vi "Create Group Transfers.vi"(7 "direction":T3, 8 "error in (no error)":errorcluster, 9 "Group ID":string, 10 "dsf refnum in":T2, 11 "Section Ptr":T1 format="%.0x") -> (0 "error out":errorcluster)   [LabVIEW 2017, in "Data Sharing Framework System Explorer.lvlib"]
uses:
  Data Sharing Framework System Explorer.lvlib
  dsf core/Source/DSF Configuration API/1.0.0/Public/Controls/DSF Direction.ctl
  dsf core/Source/DSF Configuration API/1.0.0/Public/Controls/DSF Config Data RefNum.ctl
  <vilib>/NI Veristand/Custom Device API/Custom Device Item Ref.ctl
  dsf core/Source/DSF Configuration API/1.0.0/Public/Read Item Child IDs/Read Group Transfer IDs.vi
  <vilib>/NI VeriStand/Custom Device API/Custom Device API.lvlib
  dsf core/Source/DSF Configuration API/1.0.0/DSF Configuration API.lvlib
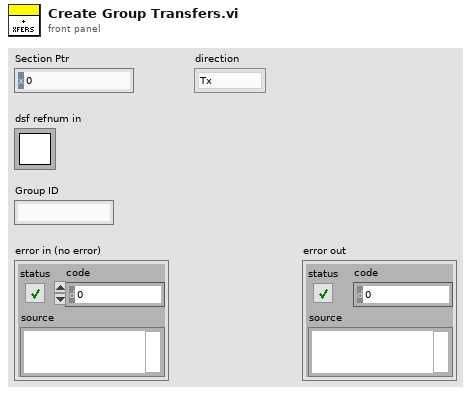
[diagram p1: front panel]
types:
  T1 = typedef "Custom Device API.lvlib/Custom Device Item Ref.ctl" = u64
  T2 = typedef "DSF Configuration API.lvlib/DSF Config Data RefNum.ctl" = refnum<k1>
  T3 = typedef "DSF Configuration API.lvlib/DSF Direction.ctl" = enum8{"Tx", "Rx"}
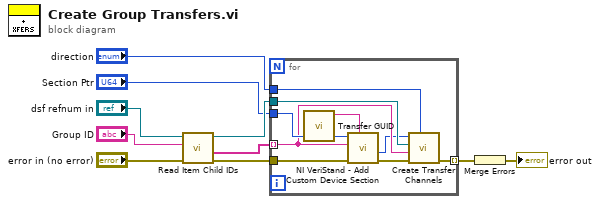
[diagram p0: block diagram]
diagram:
  n1 = call-poly "Read Item Child IDs.vi"("error in (no error)"="error in (no error)", "Group ID"="Group ID", "dsf refnum"="dsf refnum in") -> ("error out"=w3:errorcluster, "Transfer IDs"=w4:string[], "dsf refnum out"=w6:T2)  [unwired: 5 in, 1 out]
  n2 = for {
    tunnel: w4 -> [w13] mode=indexing
    tunnel: w3 -> [w19]
    tunnel: [w17] -> w2 mode=indexing
    tunnel: "Section Ptr" -> [w18]
    tunnel: w6 -> [w15]
    tunnel: "direction" -> [w14]
    n3 = call "Transfer GUID.vi"() -> ("GUID"=w11:string)  [unwired: 11 in]
    n4 = call <vilib>:"NI VeriStand - Add Custom Device Section.vi"("GUID (Default Section)"=w11, "error in (no error)"=w19, "Section Name"=w13, "Parent Ref in"=w18) -> ("error out"=w16:errorcluster, "Section Ptr"=w12:T1)  [unwired: 4 in, 2 out]
    n5 = call "Create Transfer Channels.vi"("direction"=w14, "error in (no error)"=w16, "Transfer ID"=w13, "Refnum in"=w15, "Section Ptr"=w12) -> ("error out"=w17:errorcluster)  [unwired: 6 in]
  }
  n6 = Merge Errors(w2) -> (→"error out":errorcluster)
